vi "call dll.vi"() -> ()   [LabVIEW 2015]
uses:
  Type/_Server Command.ctl
  EH-Simplicity/acquisition/Addons/Sim/Interface DLL.dll
panel:
  out "len2":i32
  out "len":i32
  out "error out":errorcluster
  out "Error":string
  out "Data":string
  in  "Message":string
  in  "Command":T1=enum."Start Run"
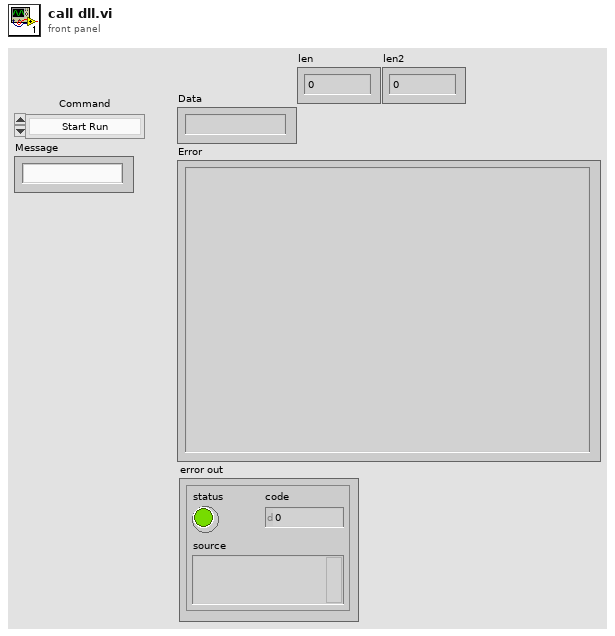
[diagram p1: front panel]
types:
  T1 = typedef "_Server Command.ctl" = enum16{"Hide Server", "Show Server", "Close Server", "Start Run", "Start Actual Run", "Stop Run", "Runtime Update", "Get Data", "Get Status", "Get Table", "Set Table", "Get Configuration", "Reserved", "Get Memory Map", "Read ADC", "Set Oscillator", "Reboot", "Backup Firmware", "Update Firmware", "Auxiliary Update", "System Status", "Start System", "Shutdown System", "Start LC Equilibration", "Get LC Status", "Get LC Configuration", "Get LC Method Contents", "Rinse Autosampler", "Pump OnOff", "Oven OnOff", "Get LC Error", "Clear LC Error", "Set LC Input Logic", "Set LC Hold Logic", "Lock Server", "Get Current Method", "Get Real Time Data", "Connect LC", "Disconnect LC"}
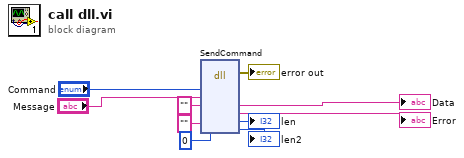
[diagram p0: block diagram]
diagram:
  w4 = 0 ("len")
  n1 = dll-call lib="D:/GITRepositories/Ionics/GitHub/EH-Simplicity/acquisition/Addons/Sim/Interface DLL.dll" fn="SendCommand"("Command"="Command", "Message"="Message", "Data"="", "Error"="", "len"=w4, "len2"=w4) -> (error out=→"error out":errorcluster, "Data"=→"Data":string, "Error"=→"Error":string, "len"=→"len":i32, "len2"=→"len2":i32)  [unwired: 6 in, 1 out]
